vi "Determine Warnings 3-9.vi"() -> ()   [LabVIEW 2014]
panel:
  in  "Max Wind Speed":dbl
  in  "Current Wind Speed":dbl
  out "Warning Text":string
  out "Warning?":bool
  out "Warning?":bool
  out "Warning Text":string
  in  "Min Temp":dbl
  in  "Max Temp":dbl
  in  "Current Temp":dbl
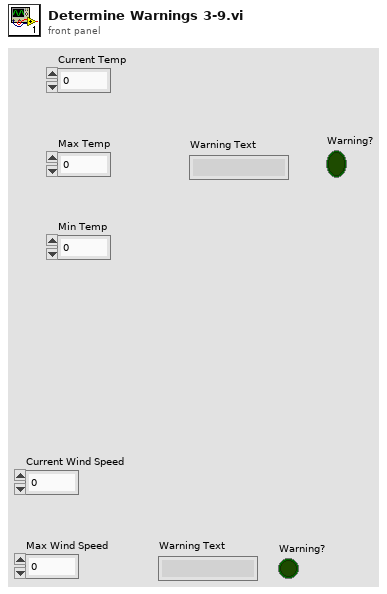
[diagram p1: front panel]
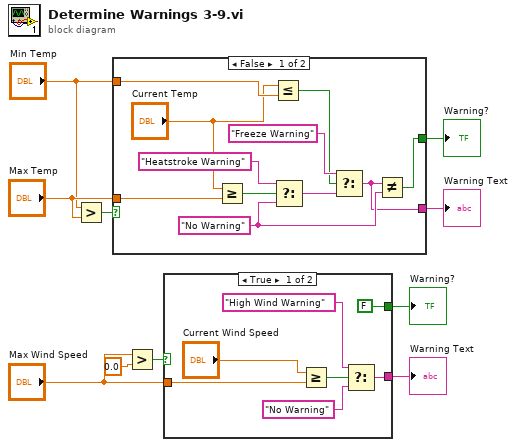
[diagram p0: block diagram]
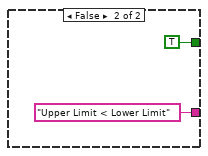
[diagram p2: hidden frame]
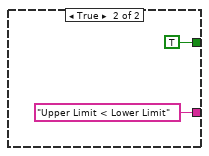
[diagram p3: hidden frame]
diagram:
  n1 = Greater?(x="Min Temp", y="Max Temp") -> (0:w8:bool)
  n2 = case shown="False" w8 {
    tunnel: "Min Temp" -> [w21 _]
    tunnel: "Max Temp" -> [w19 _]
    tunnel: [w12 TRUE] -> w7
    tunnel: [w11 "Upper Limit < Lower Limit"] -> w6
    frame False {
      w18 = "No Warning"
      n3 = Greater Or Equal?(x="Current Temp", y=w19) -> (x >= y?=w14:bool)
      n4 = Less Or Equal?(x="Current Temp", y=w21) -> (x <= y?=w13:bool)
      n5 = Select(t="Heatstroke Warning", s=w14, f=w18) -> (s? t:f=w17:string)
      n6 = Select(t="Freeze Warning", s=w13, f=w17) -> (s? t:f=w11:string)
      n7 = Not Equal?(x=w11, y=w18) -> (x != y?=w12:bool)
    }
    frame True {
    }
  }
  "Warning Text" <- w6
  "Warning?" <- w7
  n8 = Greater?(x="Max Wind Speed", y=0.0) -> (0:w1:bool)
  n9 = case shown="True" w1 {
    tunnel: "Max Wind Speed" -> [w29 _]
    tunnel: [w25 "Upper Limit < Lower Limit"] -> w5
    tunnel: [FALSE TRUE] -> w4
    frame True {
      n10 = Greater Or Equal?(x="Current Wind Speed", y=w29) -> (x >= y?=w26:bool)
      n11 = Select(t="High Wind Warning", s=w26, f="No Warning") -> (s? t:f=w25:string)
    }
    frame False {
    }
  }
  "Warning Text" <- w5
  "Warning?" <- w4
